vi "Joystick_Controlled_PWM_r0.vi"() -> ()   [LabVIEW 2015]
uses:
  <vilib>/myRIO/Instrument Drivers/Onboard IO/PWM/typedefs/PWM Reference.ctl
  <vilib>/myRIO/Common/Instrument Driver Framework/Utilities/typedefs/myRIO Generic Hardware Reference.ctl
  <vilib>/myRIO/Common/Instrument Driver Framework/Utilities/typedefs/Hardware Version Enum.ctl
  <vilib>/myRIO/Common/Instrument Driver Framework/Utilities/typedefs/myRIO v1.0 Reference.ctl
  <vilib>/myRIO/Common/Instrument Driver Framework/Utilities/typedefs/Generic FPGA Reference.ctl
  <vilib>/myRIO/Common/Instrument Driver Framework/myRIO v1.0/PWM/typedefs/PWM Channels Enum.ctl
  <vilib>/myRIO/Instrument Drivers/Onboard IO/PWM/typedefs/PWM Configuration.ctl
  <vilib>/userdefined/High Color/nirio_resource_hc.ctl
  <vilib>/myRIO/Common/Instrument Driver Framework/myRIO v1.0/PWM/vis/myRIO v1.1 Open PWM.vi
  <vilib>/myRIO/Common/Instrument Driver Framework/Utilities/vis/Validate Channels.vi
  <vilib>/myRIO/Common/Instrument Driver Framework/myRIO v1.0/PWM/vis/myRIO v1.0 Reserve PWM.vi
  <vilib>/myRIO/Common/Instrument Driver Framework/myRIO v1.0/PWM/vis/myRIO v1.0 Close PWM.vi
  <vilib>/myRIO/Common/Instrument Driver Framework/myRIO v1.0/PWM/vis/myRIO v1.0 Build MUX Configuration PWM.vi
  <vilib>/myRIO/Common/Instrument Driver Framework/myRIO v1.0/Resource Manager/vis/myRIO v1.0 Reserve Channel List.vi
  <vilib>/myRIO/Common/Instrument Driver Framework/myRIO v1.0/PWM/vis/myRIO v1.0 Unreserve PWM.vi
  <vilib>/myRIO/Common/Instrument Driver Framework/myRIO v1.0/Resource Manager/vis/myRIO v1.0 Create Configuration List.vi
  <vilib>/myRIO/Common/Instrument Driver Framework/myRIO v1.0/Resource Manager/vis/myRIO v1.0 Reserve Channel.vi
  <vilib>/myRIO/Common/Instrument Driver Framework/myRIO v1.0/Resource Manager/vis/myRIO v1.0 Unreserve Channel.vi
  <vilib>/myRIO/Common/Instrument Driver Framework/myRIO v1.0/Resource Manager/vis/myRIO v1.0 Unreserve Channel List.vi
  <vilib>/myRIO/Common/Instrument Driver Framework/myRIO v1.0/Resource Manager/vis/myRIO v1.0 Build Mutex Name.vi
  <vilib>/Utility/VariantDataType/GetNumericInfo.vi
  <vilib>/Utility/error.llb/Error Cluster From Error Code.vi
  <vilib>/myRIO/Common/Instrument Driver Framework/myRIO v1.0/myRIO v1.1 Open.vi
  <vilib>/myRIO/Common/Instrument Driver Framework/Utilities/vis/IO Manager.vi
  <vilib>/myRIO/Common/Instrument Driver Framework/Utilities/vis/Configuration Manager.vi
  <vilib>/myRIO/Common/Instrument Driver Framework/myRIO v1.0/Resource Manager/vis/myRIO v1.0 Configure IO.vi
  <vilib>/myRIO/Common/Instrument Driver Framework/myRIO v1.0/myRIO v1.0 Close.vi
  <vilib>/myRIO/Common/Instrument Driver Framework/myRIO v1.0/PWM/vis/myRIO v1.0 Write PWM.vi
  <vilib>/myRIO/Common/Instrument Driver Framework/myRIO v1.0/PWM/vis/myRIO v1.0 Shutdown PWM.vi
  <vilib>/myRIO/Instrument Drivers/Onboard IO/PWM/vis/myRIO PWM Open.xnode
  <vilib>/myRIO/Instrument Drivers/Onboard IO/PWM/PWM.lvlib
panel:
  out "Right Duty Cycle":dbl
  out "Left Duty Cycle":dbl
  in  "stop":bool
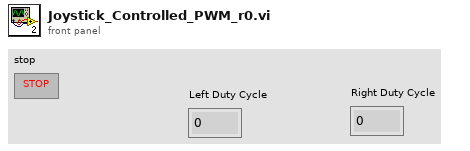
[diagram p1: front panel]
types:
  T1 = typedef "nirio_resource_hc.ctl" = tag
  T2 = typedef "Hardware Version Enum.ctl" = enum16{"Unknown", "myRIO-1900", "myRIO-1950", "roboRIO"}
  T3 = typedef "PWM.lvlib/PWM Reference.ctl" = cluster{"myRIO Reference":T4, "PWM Channels Enum":T7, "PWM Configuration":T8}
  T4 = typedef "myRIO Generic Hardware Reference.ctl" = cluster{"myRIO Model":T2, "myRIO Hardware Reference":T5}
  T5 = typedef "myRIO v1.0 Reference.ctl" = cluster{"Generic FPGA Reference":T6, "Allow multiple opens":bool}
  T6 = typedef "Generic FPGA Reference.ctl" = refnum<k20>
  T7 = typedef "PWM Channels Enum.ctl" = enum16{"Not Connected", "C/PWM0", "C/PWM1", "A/PWM0", "A/PWM1", "A/PWM2", "B/PWM0", "B/PWM1", "B/PWM2", "PWM/PWM0", "PWM/PWM1", "PWM/PWM2", "PWM/PWM3", "PWM/PWM4", "PWM/PWM5", "PWM/PWM6", "PWM/PWM7", "PWM/PWM8", "PWM/PWM9"}
  T8 = typedef "PWM.lvlib/PWM Configuration.ctl" = cluster{"Frequency":dbl, "Duty Cycle":dbl}
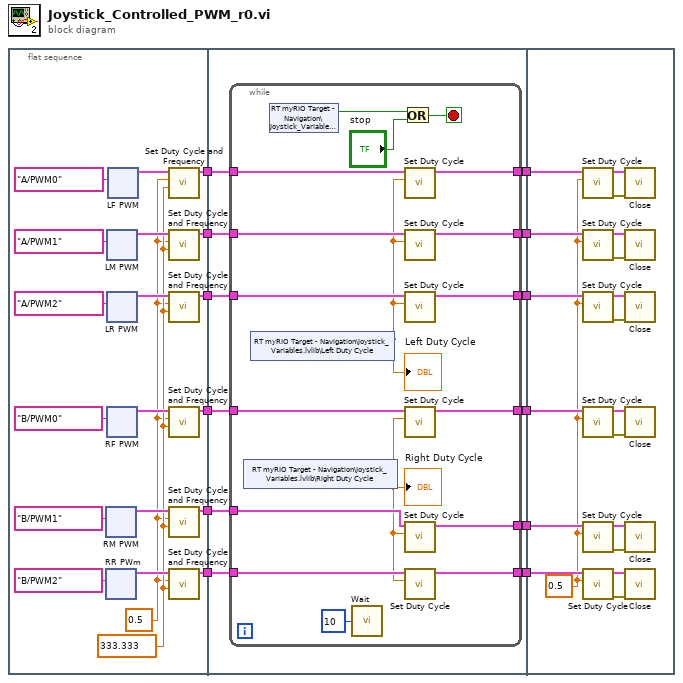
[diagram p0: block diagram]
diagram:
  n1 = flat-sequence {
    tunnel: [w18] -> w12
    tunnel: [w17] -> w11
    tunnel: [w16] -> w10
    tunnel: [w15] -> w9
    tunnel: [w14] -> w8
    tunnel: [w13] -> w7
    tunnel: w12 -> [w140]
    tunnel: w11 -> [w139]
    tunnel: w10 -> [w138]
    tunnel: w9 -> [w137]
    tunnel: w8 -> [w136]
    tunnel: w7 -> [w135]
    tunnel: [w134] -> w6
    tunnel: [w133] -> w5
    tunnel: [w132] -> w4
    tunnel: [w131] -> w3
    tunnel: [w130] -> w2
    tunnel: [w129] -> w1
    tunnel: w6 -> [w177]
    tunnel: w5 -> [w176]
    tunnel: w4 -> [w175]
    tunnel: w3 -> [w174]
    tunnel: w2 -> [w173]
    tunnel: w1 -> [w172]
    frame #0 {
      w19 = 0.5
      w20 = 333.333
      n2 = xnode "RM PWM"("Channel Name"=tag "B/PWM1") -> ("PWM Ref Out"=w22:T3)  [unwired: 2 in, 1 out]
      n3 = xnode "RR PWm"("Channel Name"=tag "B/PWM2") -> ("PWM Ref Out"=w21:T3)  [unwired: 2 in, 1 out]
      n4 = xnode "LM PWM"("Channel Name"=tag "A/PWM1") -> ("PWM Ref Out"=w25:T3)  [unwired: 2 in, 1 out]
      n5 = xnode "LR PWM"("Channel Name"=tag "A/PWM2") -> ("PWM Ref Out"=w24:T3)  [unwired: 2 in, 1 out]
      n6 = xnode "RF PWM"("Channel Name"=tag "B/PWM0") -> ("PWM Ref Out"=w23:T3)  [unwired: 2 in, 1 out]
      n7 = xnode "LF PWM"("Channel Name"=tag "A/PWM0") -> ("PWM Ref Out"=w26:T3)  [unwired: 2 in, 1 out]
      n8 = call <vilib>:"Set Duty Cycle and Frequency.vi"("Frequency [Hz]"=w20, "Duty Cycle"=w19, "PWM Ref In"=w26) -> ("PWM Ref Out"=w18:T3)  [unwired: 6 in, 1 out]
      n9 = call <vilib>:"Set Duty Cycle and Frequency.vi"("Frequency [Hz]"=w20, "Duty Cycle"=w19, "PWM Ref In"=w25) -> ("PWM Ref Out"=w17:T3)  [unwired: 6 in, 1 out]
      n10 = call <vilib>:"Set Duty Cycle and Frequency.vi"("Frequency [Hz]"=w20, "Duty Cycle"=w19, "PWM Ref In"=w24) -> ("PWM Ref Out"=w16:T3)  [unwired: 6 in, 1 out]
      n11 = call <vilib>:"Set Duty Cycle and Frequency.vi"("Frequency [Hz]"=w20, "Duty Cycle"=w19, "PWM Ref In"=w23) -> ("PWM Ref Out"=w15:T3)  [unwired: 6 in, 1 out]
      n12 = call <vilib>:"Set Duty Cycle and Frequency.vi"("Frequency [Hz]"=w20, "Duty Cycle"=w19, "PWM Ref In"=w22) -> ("PWM Ref Out"=w14:T3)  [unwired: 6 in, 1 out]
      n13 = call <vilib>:"Set Duty Cycle and Frequency.vi"("Frequency [Hz]"=w20, "Duty Cycle"=w19, "PWM Ref In"=w21) -> ("PWM Ref Out"=w13:T3)  [unwired: 6 in, 1 out]
    }
    frame #1 {
      n14 = while {
        tunnel: w140 -> [w158]
        tunnel: w139 -> [w157]
        tunnel: w138 -> [w156]
        tunnel: w137 -> [w155]
        tunnel: w136 -> [w154]
        tunnel: w135 -> [w153]
        tunnel: [w151] -> w134
        tunnel: [w150] -> w133
        tunnel: [w149] -> w132
        tunnel: [w148] -> w131
        tunnel: [w147] -> w130
        tunnel: [w146] -> w129
        stop <- w145 stop-if-true
        n15 = shared-variable "RT myRIO Target - Navigation\\Joystick_Variables.lvlib\\Right Duty Cycle"() -> (w142:dbl)  [unwired: 1 in, 1 out]
        "Right Duty Cycle" <- w142
        n16 = shared-variable "RT myRIO Target - Navigation\\Joystick_Variables.lvlib\\Left Duty Cycle"() -> (w141:dbl)  [unwired: 1 in, 1 out]
        "Left Duty Cycle" <- w141
        n17 = shared-variable "RT myRIO Target - Navigation\\Joystick_Variables.lvlib\\Dig"() -> (w144:bool)  [unwired: 1 in, 1 out]
        n18 = call "Wait"("Count(mSec)"=u32 10) -> ()  [unwired: 1 out]
        n19 = Or(x=w144, y="stop") -> (x .or. y?=w145:bool)
        n20 = call <vilib>:"Set Duty Cycle.vi"("Duty Cycle"=w141, "PWM Ref In"=w158) -> ("PWM Ref Out"=w151:T3)  [unwired: 7 in, 1 out]
        n21 = call <vilib>:"Set Duty Cycle.vi"("Duty Cycle"=w141, "PWM Ref In"=w157) -> ("PWM Ref Out"=w150:T3)  [unwired: 7 in, 1 out]
        n22 = call <vilib>:"Set Duty Cycle.vi"("Duty Cycle"=w141, "PWM Ref In"=w156) -> ("PWM Ref Out"=w149:T3)  [unwired: 7 in, 1 out]
        n23 = call <vilib>:"Set Duty Cycle.vi"("Duty Cycle"=w142, "PWM Ref In"=w155) -> ("PWM Ref Out"=w148:T3)  [unwired: 7 in, 1 out]
        n24 = call <vilib>:"Set Duty Cycle.vi"("Duty Cycle"=w142, "PWM Ref In"=w154) -> ("PWM Ref Out"=w147:T3)  [unwired: 7 in, 1 out]
        n25 = call <vilib>:"Set Duty Cycle.vi"("Duty Cycle"=w142, "PWM Ref In"=w153) -> ("PWM Ref Out"=w146:T3)  [unwired: 7 in, 1 out]
      }
    }
    frame #2 {
      w159 = 0.5
      n26 = call <vilib>:"Set Duty Cycle.vi"("Duty Cycle"=w159, "PWM Ref In"=w177) -> ("error out"=w171:errorcluster, "PWM Ref Out"=w170:T3)  [unwired: 7 in]
      n27 = call <vilib>:"Set Duty Cycle.vi"("Duty Cycle"=w159, "PWM Ref In"=w176) -> ("error out"=w169:errorcluster, "PWM Ref Out"=w168:T3)  [unwired: 7 in]
      n28 = call <vilib>:"Set Duty Cycle.vi"("Duty Cycle"=w159, "PWM Ref In"=w175) -> ("error out"=w167:errorcluster, "PWM Ref Out"=w166:T3)  [unwired: 7 in]
      n29 = call <vilib>:"Set Duty Cycle.vi"("Duty Cycle"=w159, "PWM Ref In"=w174) -> ("error out"=w165:errorcluster, "PWM Ref Out"=w164:T3)  [unwired: 7 in]
      n30 = call <vilib>:"Set Duty Cycle.vi"("Duty Cycle"=w159, "PWM Ref In"=w173) -> ("error out"=w163:errorcluster, "PWM Ref Out"=w162:T3)  [unwired: 7 in]
      n31 = call <vilib>:"Set Duty Cycle.vi"("Duty Cycle"=w159, "PWM Ref In"=w172) -> ("error out"=w161:errorcluster, "PWM Ref Out"=w160:T3)  [unwired: 7 in]
      n32 = call <vilib>:"Close.vi"("error in (no error)"=w171, "PWM Ref In"=w170) -> ()  [unwired: 9 in, 1 out]
      n33 = call <vilib>:"Close.vi"("error in (no error)"=w169, "PWM Ref In"=w168) -> ()  [unwired: 9 in, 1 out]
      n34 = call <vilib>:"Close.vi"("error in (no error)"=w167, "PWM Ref In"=w166) -> ()  [unwired: 9 in, 1 out]
      n35 = call <vilib>:"Close.vi"("error in (no error)"=w165, "PWM Ref In"=w164) -> ()  [unwired: 9 in, 1 out]
      n36 = call <vilib>:"Close.vi"("error in (no error)"=w163, "PWM Ref In"=w162) -> ()  [unwired: 9 in, 1 out]
      n37 = call <vilib>:"Close.vi"("error in (no error)"=w161, "PWM Ref In"=w160) -> ()  [unwired: 9 in, 1 out]
    }
  }
